vi "GT Set Stop Io.vi"(6 "inputIndex":i16, 7 "inputType":i16, 8 "error in (no error)":errorcluster caption="错误输入（无错误）", 9 "stopType":i16, 10 "axis":i16, 11 "cardNum":i16) -> (0 "error out":errorcluster caption="错误输出", 3 "function return":i16)   [LabVIEW 2014, in "gts.lvlib"]
doc: "GT_API GT_SetStopIo(short cardNum,short axis,short stopType,short inputType,short inputIndex);"
uses:
  gts.lvlib
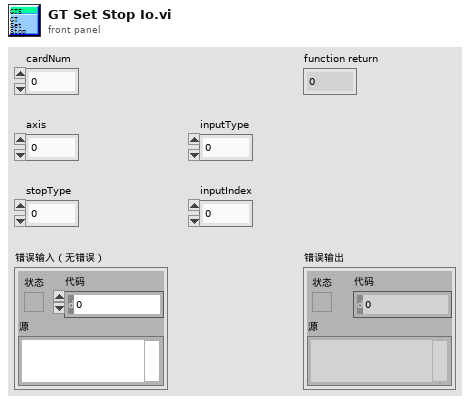
[diagram p1: front panel]
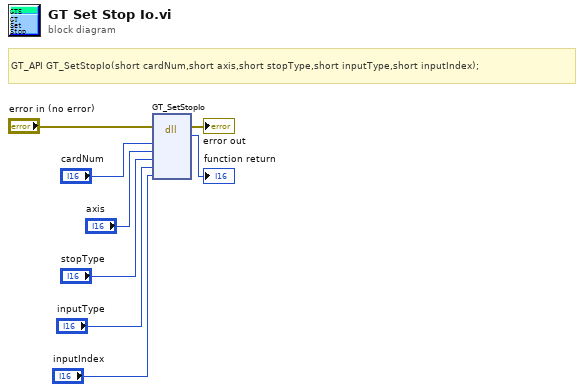
[diagram p0: block diagram]
diagram:
  # "GT_API GT_SetStopIo(short cardNum,short axis,short stopType,short inputType,short inputIndex);"
  n1 = dll-call lib="PTH2habs D固高科技资料GTS控制卡GTS卡18年上半年资料dllVC32bit\nmulti_cardgts.*" fn="GT_SetStopIo"(error in="error in (no error)", "cardNum"="cardNum", "axis"="axis", "stopType"="stopType", "inputType"="inputType", "inputIndex"="inputIndex") -> (error out=→"error out":errorcluster, →"function return":i16)  [unwired: 7 in, 1 out]
